vi "mod_Resample (complex) v2.vi"(0 "x":cdb[](array[numeric]) format="%.2f", 5 "config":T1={"new sample period"=0.0, "Timing Jitter"=enum."Interpolation", "first point location"=0.0, "prototype filter"={"h"=[], "Max Decimation"=1024.0}} {"prototype filter"."h" format="%.2f"; "prototype filter"."Max Decimation" format="%.2f"; "first point location" format="%.2f"; "new sample period" format="%.2f"}, 13 "Reset? (T)":bool=TRUE) -> (4 "y":cdb[](array[numeric]) format="%.2f", 15 "error out":errorcluster)   [LabVIEW 2020, in "niAMT.lvlib"]
uses:
  <vilib>/addons/Modulation/niAMT.lvlib
  nilvamt.dll
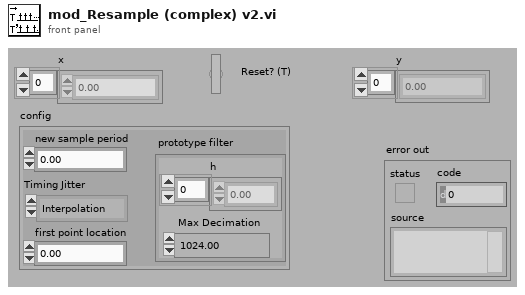
[diagram p1: front panel]
types:
  T1 = cluster{"new sample period":dbl, "Timing Jitter":enum32{"Interpolation", "Rounding"}, "first point location":dbl, "prototype filter":cluster{"h":dbl[], "Max Decimation":dbl}}
  T2 = cluster{"precondition":cdb[], "preconditionLen":i32, "extractFilterBuffer":dbl[], "scaling":dbl, "extractFilterLeftLen":i32, "extractFilterRightLen":i32, "method":i32, "new sample period":dbl, "offset":dbl, "index":i32}
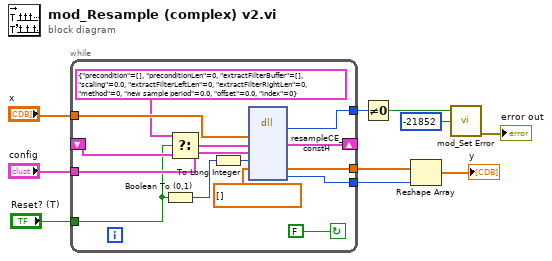
[diagram p0: block diagram]
diagram:
  n1 = while {
    tunnel: "Reset? (T)" -> [w14]
    tunnel: "config" -> [w19]
    tunnel: [w20] -> w7
    tunnel: [w21] -> w9
    shift-left: _ -> [w17]
    shift-right: [w16] -> _
    tunnel: "x" -> [w23]
    tunnel: [w11] -> w4
    stop <- FALSE continue-if-true
    n2 = Boolean To (0,1)(Boolean=w14) -> (0, 1=w13:i16)
    n3 = Select(t=T2 {"precondition"=[], "preconditionLen"=0, "extractFilterBuffer"=[], "scaling"=0.0, "extractFilterLeftLen"=0, "extractFilterRightLen"=0, "method"=0, "new sample period"=0.0, "offset"=0.0, "index"=0} ("state"), s=w14, f=w17) -> (s? t:f=w18:T2)
    n4 = To Long Integer(number=w13) -> (32bit integer=w12:i32)
    n5 = dll-call lib="nilvamt.*" fn="resampleCE_constH"("xH"=w23, "state"=w18, "config"=w19, "reset"=w12, "yH"=cdb[] [] ("y")) -> ("return type"=w11:i32, "state"=w16:T2, "yH"=w21:cdb[], "out_len"=w20:i32)  [unwired: 6 in, 3 out]
  }
  n6 = Not Equal To 0?(x=w4) -> (x != 0?=w3:bool)
  n7 = Reshape Array(w9, w7) -> (→"y":cdb[])
  n8 = call <vilib>:"mod_Set Error.vi"("code"=-21852, "status"=w3) -> ("error out"=→"error out":errorcluster)  [unwired: 6 out]
